vi "Configure X Scale.vi"(6 "X Reference Value (0 s)":dbl, 8 "error in (no error)":errorcluster, 9 "Manual Scale Per Division (1)":dbl=1.0, 10 "Auto X Scaling (T: Enable)":bool=TRUE, 11 "VISA resource name":refnum<visa-resource-name>) -> (0 "error out":errorcluster, 3 "VISA resource name out":refnum<visa-resource-name>)   [LabVIEW 2014, in "Agilent MXA Series.lvlib"]
doc: "Sets the scale and reference value of X axis.\n\nYou can use this VI only under Burst Power, Power Stat CCDF measurement types."
uses:
  Agilent MXA Series.lvlib
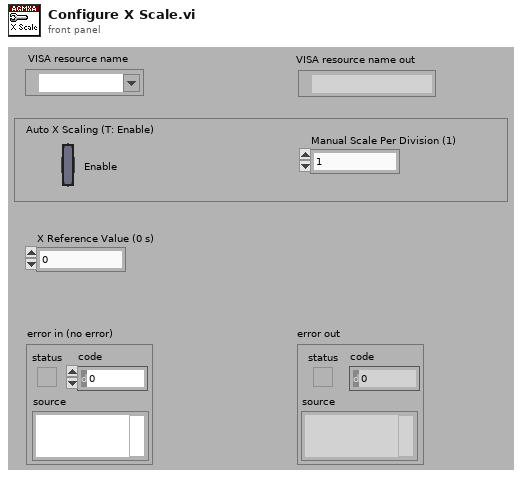
[diagram p1: front panel]
types:
  T1 = typedef "Agilent MXA Series.lvlib/Extended User Data.ctl" = cluster{"Measurement Type":i32, "Agilent MXA/EXA Model":i32}
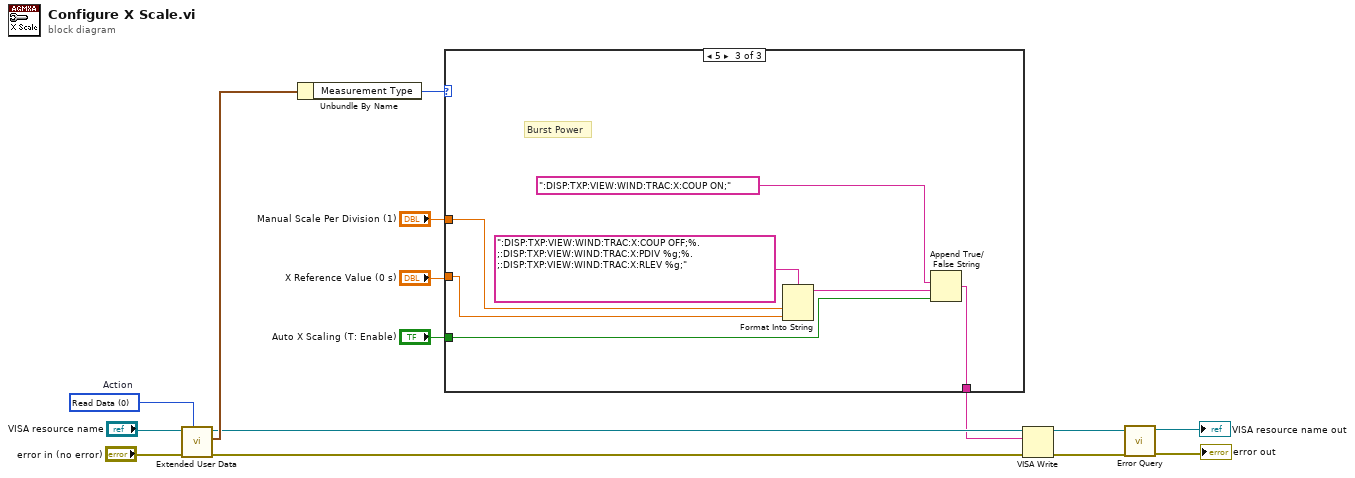
[diagram p0: block diagram]
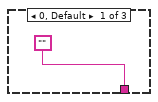
[diagram p2: hidden frame]
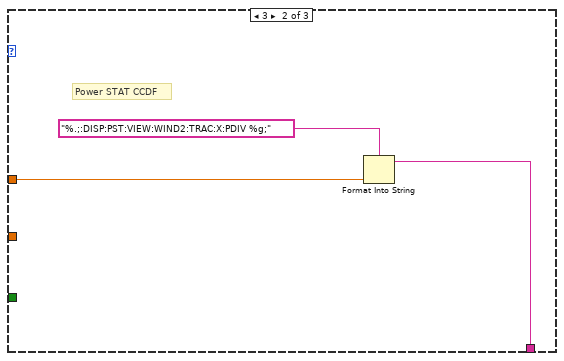
[diagram p3: hidden frame]
diagram:
  w13 = 0 items=["Read Data", "Write Data", "Clear Data", "Clear ALL Data"]  # Action
  n1 = call "Extended User Data.vi"("Action (1:Write Data)"=w13, "Error In (no error)"="error in (no error)", "VISA resource name in"="VISA resource name") -> ("Error Out"=w6:errorcluster, "User Data Out"=w12:T1, "VISA resource name out"=w7:refnum<visa-resource-name>)  [unwired: 6 in]
  n2 = Unbundle By Name(w12) -> ("Measurement Type"=w11:i32)
  n3 = case shown="5" w11 {
    tunnel: "Manual Scale Per Division (1)" -> [_ w18 w22]
    tunnel: "X Reference Value (0 s)" -> [_ _ w21]
    tunnel: "Auto X Scaling (T: Enable)" -> [_ _ w26]
    tunnel: ["" w17 w25] -> w1
    frame 0, Default {
    }
    frame 3 {
      # "Power STAT CCDF"
      n4 = Format Into String(format string="%.;:DISP:PST:VIEW:WIND2:TRAC:X:PDIV %g;", w18) -> (resulting string=w17:string)  [unwired: 2 in, 1 out]
    }
    frame 5 {
      # "Burst Power"
      n5 = Format Into String(format string=":DISP:TXP:VIEW:WIND:TRAC:X:COUP OFF;%.;:DISP:TXP:VIEW:WIND:TRAC:X:PDIV %g;%.;:DISP:TXP:VIEW:WIND:TRAC:X:RLEV %g;", w22, w21) -> (resulting string=w20:string)  [unwired: 2 in, 1 out]
      n6 = Append True/False String(1:w26, 2:w20, 3:":DISP:TXP:VIEW:WIND:TRAC:X:COUP ON;") -> (0:w25:string)  [unwired: 1 in]
    }
  }
  n7 = VISA Write(VISA resource name=w7, write buffer=w1, error in (no error)=w6) -> (VISA resource name out=w4:refnum<visa-resource-name>, error out=w5:errorcluster)  [unwired: 1 out]
  n8 = call "Error Query.vi"("error in (no error)"=w5, "VISA resource name"=w4) -> ("error out"=→"error out":errorcluster, "VISA resource name out"=→"VISA resource name out":refnum<visa-resource-name>)  [unwired: 6 in, 2 out]
